vi "Drag & Drop End Single.vi"(8 "errorin":errorcluster, 11 "References In":T1) -> (0 "error out":errorcluster)   [LabVIEW 2015]
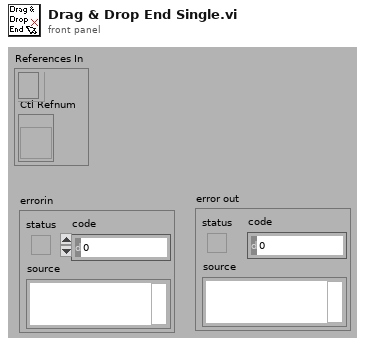
[diagram p1: front panel]
types:
  T1 = cluster{"Event Registration Refnum":refnum<event-registration>, "Ctl Refnum":refnum<vi>}
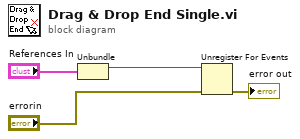
[diagram p0: block diagram]
diagram:
  n1 = Unbundle("References In") -> ("Event Registration Refnum"=w4:refnum<event-registration>)  [unwired: 1 out]
  n2 = Unregister For Events(event registration refnum=w4, error in="errorin") -> (error out=→"error out":errorcluster)
